vi "Get Handle Messages VI Reference.vi"(8 "error in (no error)":errorcluster, 11 "Getter Generator in":refnum<class "Getter Generator.lvclass">) -> (0 "error out":errorcluster, 3 "Getter Generator out":refnum<class "Getter Generator.lvclass">)   [LabVIEW 2020, in "Method Generation.lvlib" / "Getter Generator.lvclass"]
uses:
  Getter Generator.lvclass
  Getter Generator.lvclass/Getter Generator.ctl
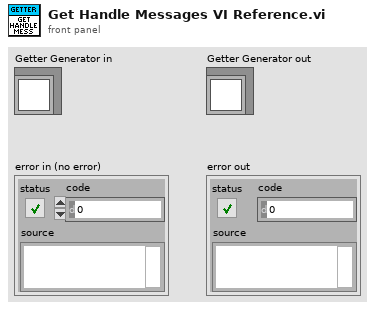
[diagram p1: front panel]
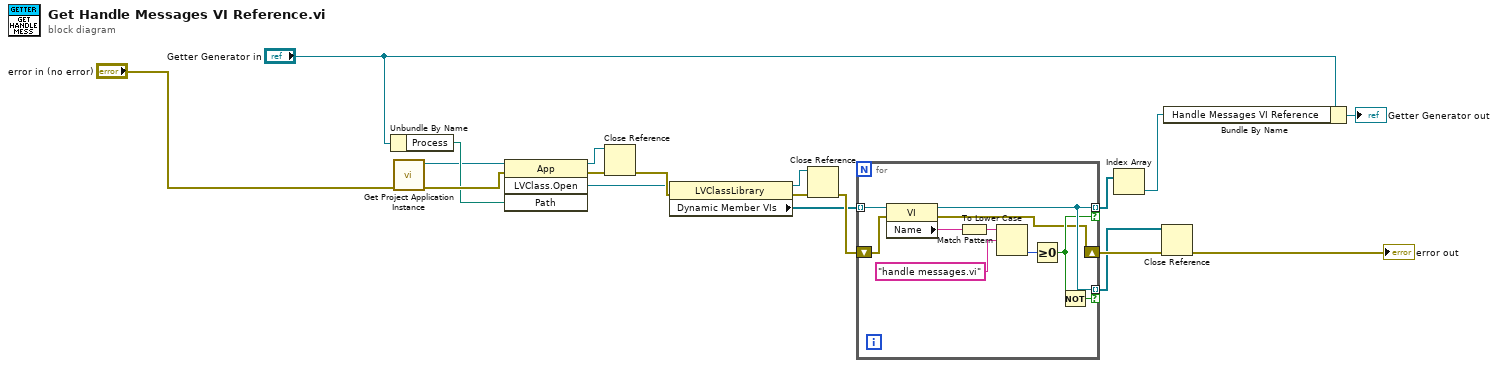
[diagram p0: block diagram]
diagram:
  n1 = Unbundle By Name("Getter Generator in") -> ("Process"=w4:path)
  n2 = call "Get Project Application Instance.vi"("error in (no error)"="error in (no error)") -> ("error out"=w5:errorcluster, "Application out"=w3:refnum<vi>)  [unwired: 9 in]
  n3 = invoke class="App" method="LVClass.Open"(reference=w3, error in=w5, "Path"=w4) -> (reference out=w7:refnum<vi>, error out=w8:errorcluster, "LVClass.Open"=w9:refnum<vi>)  [unwired: 1 in, 1 out]
  n4 = Close Reference(reference=w7, error in (no error)=w8) -> (error out=w10:errorcluster)
  n5 = property class="LVClassLibrary"(reference=w9, error in=w10) -> (reference out=w15:refnum<vi>, error out=w12:errorcluster, "Dynamic Member VIs"=w11:refnum<vi>[])
  n6 = Close Reference(reference=w15, error in (no error)=w12) -> (error out=w14:errorcluster)
  n7 = for {
    tunnel: w11 -> [w29] mode=indexing
    tunnel: [w23] -> w2 mode=indexing if=w22
    tunnel: [w23] -> w1 mode=indexing if=w21
    shift-right: [w20] -> w16
    shift-left: w14 -> [w27]
    n8 = property class="VI"(reference=w29, error in=w27) -> (reference out=w23:refnum<vi>, error out=w20:errorcluster, "Name"=w28:string)
    n9 = To Lower Case(string=w28) -> (all lower case string=w26:string)
    n10 = Match Pattern(string=w26, regular expression="handle messages.vi") -> (offset past match=w24:i32)  [unwired: 1 in, 3 out]
    n11 = Greater Or Equal To 0?(x=w24) -> (x >= 0?=w22:bool)
    n12 = Not(x=w22) -> (.not. x?=w21:bool)
  }
  n13 = Index Array(array=w2) -> (element=w17:refnum<vi>)  [unwired: 1 in]
  n14 = Close Reference(reference=w1, error in (no error)=w16) -> (error out=→"error out":errorcluster)
  n15 = Bundle By Name(cluster="Getter Generator in", "Handle Messages VI Reference"=w17) -> (→"Getter Generator out":refnum<class "Getter Generator.lvclass">)
